vi "test.vi"() -> ()   [LabVIEW 2018]
panel:
  out "字符串":string
  in  "数值":dbl
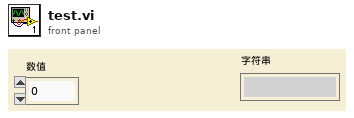
[diagram p1: front panel]
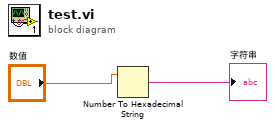
[diagram p0: block diagram]
diagram:
  n1 = Number To Hexadecimal String(2:"数值") -> (0:→"字符串":string)  [unwired: 1 in]
